vi "Remove from Parent Priv.vi"(8 "Error In":errorcluster, 9 "Unique ID":string, 10 "Parent ID":string, 11 "Tree Dictionary":variant) -> (0 "Error Out":errorcluster, 3 "Tree Dictionary Out":variant)   [LabVIEW 2017, in "Tree API.lvlib" / "Tree.lvclass"]
uses:
  Tree.lvclass
  Typedefs/Tree Cluster.ctl
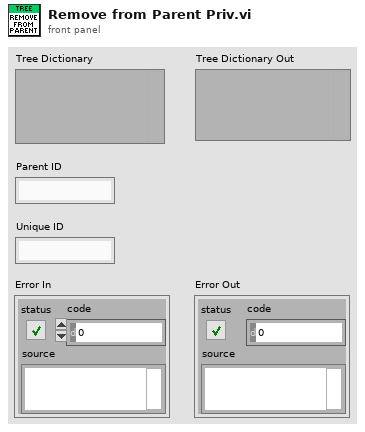
[diagram p1: front panel]
types:
  T1 = typedef "Tree API.lvlib/Tree.lvclass/Tree Cluster.ctl" = cluster{"Unique ID":string, "Parent ID":string, "Child IDs":string[], "Name":string, "MetaData":string, "Data IDs":string[]}
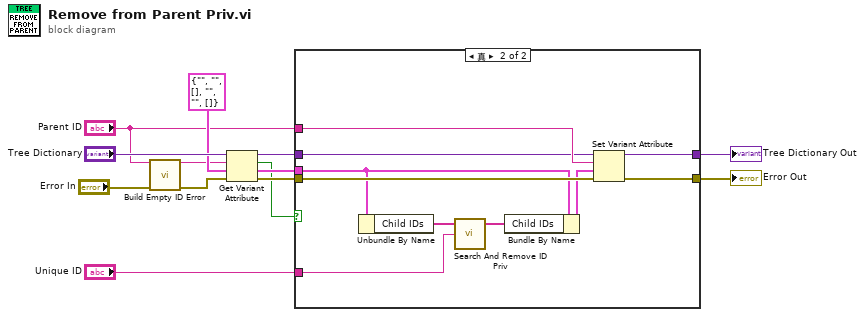
[diagram p0: block diagram]
diagram:
  n1 = call "Build Empty ID Error.vi"("Unique ID"="Parent ID", "Error In"="Error In") -> ("Unique ID Out"=w4:string, "Error Out"=w1:errorcluster)  [unwired: 12 in]
  n2 = Get Variant Attribute(Variant="Tree Dictionary", name=w4, default value (empty Variant)=T1 {"Unique ID"="", "Parent ID"="", "Child IDs"=[], "Name"="", "MetaData"="", "Data IDs"=[]} ("Cluster of class private data"), error in=w1) -> (duplicate Variant=w9:variant, found=w6:bool, value=w8:T1, error out=w10:errorcluster)
  n3 = case shown="真" w6 {
    tunnel: [w15 w25] -> w13
    tunnel: "Unique ID" -> [_ w24]
    tunnel: [w14 w23] -> w11
    tunnel: w10 -> [w14 w22]
    tunnel: "Parent ID" -> [_ w21]
    tunnel: w9 -> [w15 w19]
    tunnel: w8 -> [_ w18]
    frame False {
      # "This child had no parent before. This is normal when creating\nand adding new children. Do nothing."
    }
    frame True {
      n4 = Unbundle By Name(w18) -> ("Child IDs"=w16:string[])
      n5 = call "Search And Remove ID Priv.vi"("Remove String"=w24, "Strings In"=w16) -> ("Strings Out"=w17:string[])  [unwired: 3 in]
      n6 = Bundle By Name(cluster=w18, "Child IDs"=w17) -> (w20:T1)
      n7 = Set Variant Attribute(Variant=w19, name=w21, value=w20, error in=w22) -> (Variant out=w25:variant, error out=w23:errorcluster)  [unwired: 1 out]
    }
  }
  "Tree Dictionary Out" <- w13
  "Error Out" <- w11
